vi "system_ReadConfigure.vi"(8 "error in (no error)":errorcluster) -> (0 "error out":errorcluster, 3 "Config":T1)   [LabVIEW 2013, in "0_SystemCOnfiguration.lvlib"]
uses:
  0_SystemCOnfiguration.lvlib
  system_Config.ctl
  2_Control/ProductType.ctl
  2_Control/PathControl.ctl
panel:
  # "Function Configuration"
  # "Temprary Configuration"
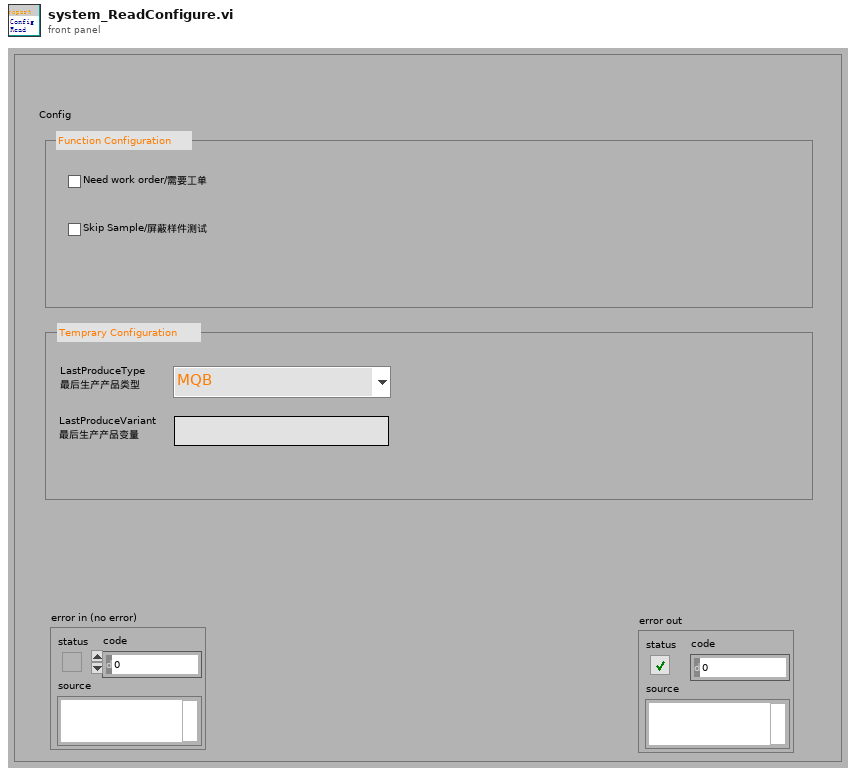
[diagram p1: front panel]
types:
  T1 = typedef "0_SystemCOnfiguration.lvlib/system_Config.ctl" = cluster{"Need work order":bool, "LastTestVariant":string, "Skip Sample":bool, "LastTestType":T2}
  T2 = typedef "ProductType.ctl" = enum16{"MQB", "Geely", "Volvo"}
  T3 = typedef "PathControl.ctl" = enum16{"UI_Banner_Path", "UI_Banner_Path1", "UI_Banner_Path2", "UI_Banner_Path0", "Menu_Manager_Run", "Menu_Debug", "Menu_Operater", "Path_ConfigFolder", "Path_Settings", "Path_Limits", "Path_TestItems", "Path_Company_logo", "Path_UUT", "Path_Customer_logo", "Path_Log_Folder", "Path_Log_Single_Folder", "Path_Config_DB", "Path_TestItem", "Path_TestLimit_Head", "Path_Log_Template", "Path_ExcelLog_Template", "Path_Label", "Path_Manual_Lable", "Path_Manual_TypeConfig", "Path_Message", "Path_ErrorLog_Folder"}
  T4 = typedef "system_Config.ctl" = cluster{"Need work order":bool, "LastTestVariant":string, "Skip Sample":bool, "LastTestType":T2}
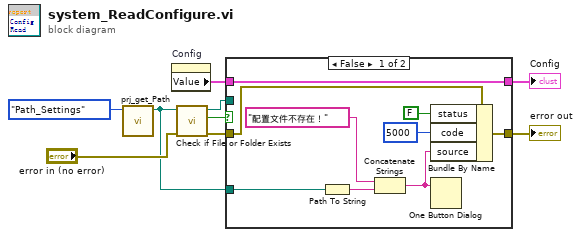
[diagram p0: block diagram]
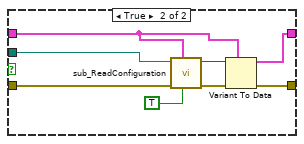
[diagram p2: hidden frame]
diagram:
  n1 = call "prj_get_Path.vi"("Path_Item"=PathControl."Path_Settings") -> ("Detail path"=w2:path)  [unwired: 10 in]
  n2 = property on="Config" class="Clust (strict)"() -> ("Value"=w3:T4)  [unwired: 2 in, 2 out]
  n3 = call <vilib>:"Check if File or Folder Exists.vi"("error in (no error)"="error in (no error)", "path"=w2) -> ("error out"=w7:errorcluster, "file or folder exists?"=w9:bool, "dup path"=w8:path)  [unwired: 7 in]
  n4 = case shown="False" w9 {
    tunnel: w8 -> [_ w26]
    tunnel: w7 -> [w17 w25]
    tunnel: [w18 w22] -> w6
    tunnel: w3 -> [w18 w20]
    tunnel: [w16 w21] -> w5
    tunnel: w2 -> [w13 _]
    frame False {
      n5 = Path To String(path=w13) -> (string=w12:string)
      n6 = Concatenate Strings("配置文件不存在！" ("消息"), w12) -> (w10:string)
      n7 = Bundle By Name(cluster=w17, "status"=FALSE, "code"=5000, "source"=w10) -> (w16:errorcluster)
      n8 = One Button Dialog(message=w10) -> ()  [unwired: 1 in, 1 out]
    }
    frame True {
      n9 = call "sub_ReadConfiguration.vi"("create file if necessary? (T)"=TRUE, "Section Formatted Cluster Type"=w20, "error in (no error)"=w25, "configuration file path"=w26) -> ("error out"=w24:errorcluster, "数据"=w23:variant)  [unwired: 6 in]
      n10 = Variant To Data(error in=w24, type=w20, Variant=w23) -> (data=w22:T4, error out=w21:errorcluster)
    }
  }
  "Config" <- w6
  "error out" <- w5
